vi "Stop Core.vi"(10 "final error code":i32, 11 "CS++BaseActor in":refnum<class "CS++BaseActor.lvclass">) -> (3 "CS++BaseActor out":refnum<class "CS++BaseActor.lvclass">)   [LabVIEW 2015, in "CS++BaseActor.lvlib" / "CS++BaseActor.lvclass"]
doc: "(<B>Filename</B>: Actor Framework.lvlib:Actor.lvclass:Stop Core.vi)\n\nDefines what the actor does before it stops. Use the <B>final error code</B> input to determine whether the actor shut down in response to an error.\n\nBy default, this method does nothing. A descendant class may override it to define behavior, such as shutting down any processes the actor initiated in its override of the Actor Core method."
uses:
  CS++BaseActor.lvclass
  CS++BaseActor.lvclass/CS++BaseActor.ctl
  Libraries/Base/Severity.ctl
  Libraries/Base/FGV Action.ctl
  <vilib>/ActorFramework/Message Enqueuer/Message Enqueuer.lvclass/Message Enqueuer.ctl
  <vilib>/ActorFramework/Message Enqueuer/Enqueue.vi
  <vilib>/ActorFramework/Message Priority Queue/Priority Enqueue.vi
  <vilib>/ActorFramework/Actor/Actor.lvclass
  <vilib>/ActorFramework/Stop Msg/Stop Msg.lvclass
  <vilib>/ActorFramework/Message Enqueuer/Message Enqueuer.lvclass
  Libraries/Base/CS++Base.lvlib
  Libraries/Utilities/CS++Utilities.lvlib
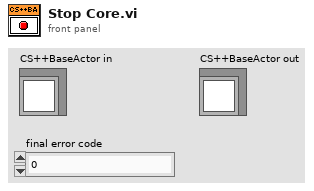
[diagram p1: front panel]
types:
  T1 = typedef "CS++Base.lvlib/FGV Action.ctl" = enum16{"add", "replace", "read", "remove", "reset", "get attributes"}
  T2 = typedef "CS++Base.lvlib/Severity.ctl" = enum16{"emergency", "alert", "critical", "error", "warning", "notice", "info", "debug"}
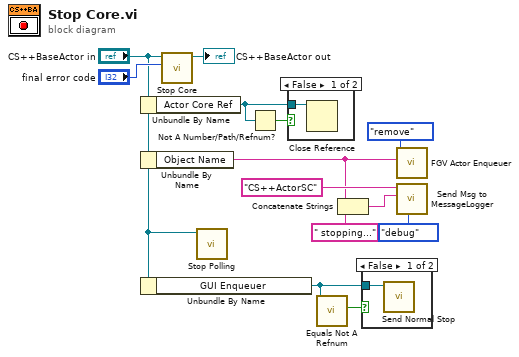
[diagram p0: block diagram]
diagram:
  n1 = Unbundle By Name("CS++BaseActor in") -> ("Actor Core Ref"=w3:refnum<vi>)
  n2 = Unbundle By Name("CS++BaseActor in") -> ("Object Name"=w5:string)
  n3 = Unbundle By Name("CS++BaseActor in") -> ("GUI Enqueuer"=w10:refnum<class "Message Enqueuer.lvclass">)
  n4 = call-parent "Stop Core.vi"("final error code"="final error code", "Actor in"="CS++BaseActor in") -> ("Actor out"=→"CS++BaseActor out":refnum<class "CS++BaseActor.lvclass">)  [unwired: 9 in]
  n5 = call "Stop Polling.vi"("CS++BaseActor in"="CS++BaseActor in") -> ()  [unwired: 9 in, 2 out]
  n6 = Not A Number/Path/Refnum?(number/path/refnum=w3) -> (NaN/Path/Refnum?=w2:bool)
  n7 = case shown="False" w2 {
    tunnel: w3 -> [w14 _]
    frame False {
      n8 = Close Reference(reference=w14) -> ()  [unwired: 1 in, 1 out]
    }
    frame True {
    }
  }
  n9 = call <vilib>:"Equals Not A Refnum.vi"("Message Enqueuer"=w10) -> ("Not a refnum?"=w9:bool)  [unwired: 10 in]
  n10 = Concatenate Strings(w5, " stopping..." ("string")) -> (w7:string)
  n11 = case shown="False" w9 {
    tunnel: w10 -> [w15 _]
    frame False {
      n12 = call <vilib>:"Send Normal Stop.vi"("Message Enqueuer"=w15) -> ()  [unwired: 10 in, 1 out]
    }
    frame True {
    }
  }
  n13 = call "FGV Actor Enqueuer.vi"("Actor Name"=w5, "Action (read)"=FGV_Action."remove") -> ()  [unwired: 5 in, 5 out]
  n14 = call "Send Msg to MessageLogger.vi"("Severity Code (info)"=Severity."debug", "Message Content"=w7, "Message Tag"="CS++ActorSC") -> ()  [unwired: 8 in, 1 out]
